vi "Boltzmann Constant.vi"() -> (2 "Boltzmann":dbl)   [LabVIEW 2015]
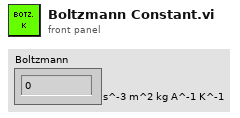
[diagram p1: front panel]
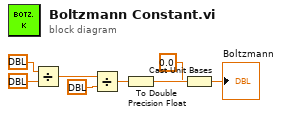
[diagram p0: block diagram]
diagram:
  n1 = Divide(x=ext[unit] 8.314472, y=ext[unit] 6.0221415e+23) -> (x/y=w5:ext[unit])
  n2 = Divide(x=w5, y=ext[unit] 1.60217652999999999996e-19) -> (x/y=w4:ext[unit])
  n3 = To Double Precision Float(number=w4) -> (double precision float=w3:dbl[unit])
  n4 = Cast Unit Bases(0:w3, 1:0.0 ("unit (none)")) -> (2:→"Boltzmann":dbl)
